vi "Scan_Table_Mode.vi"(0 "Mode":T1) -> (1 "Simulate Mode ?":bool, 2 "Log Full Res Data?":bool, 3 "Minimum Scan Period (ms)":i32)   [LabVIEW 2022 SP3]
uses:
  Anemometry/Anemometry Sub Vis/Controls/Serveds.ctl
  Anemometry/Anemometry Sub Vis/Globals/Constants_global.vi
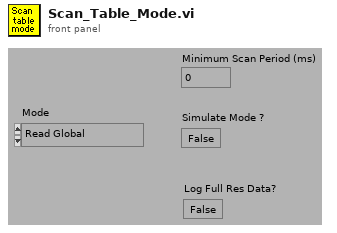
[diagram p1: front panel]
types:
  T1 = typedef "Serveds.ctl" = enum16{"Read Global", "Load Global From File"}
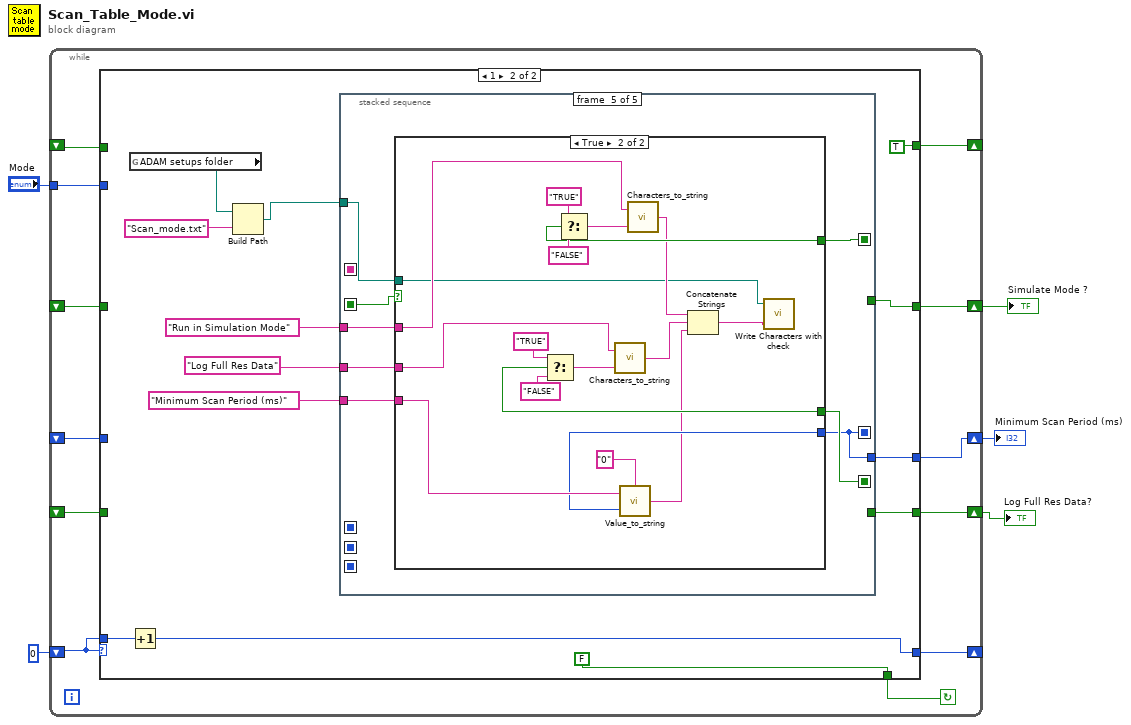
[diagram p0: block diagram]
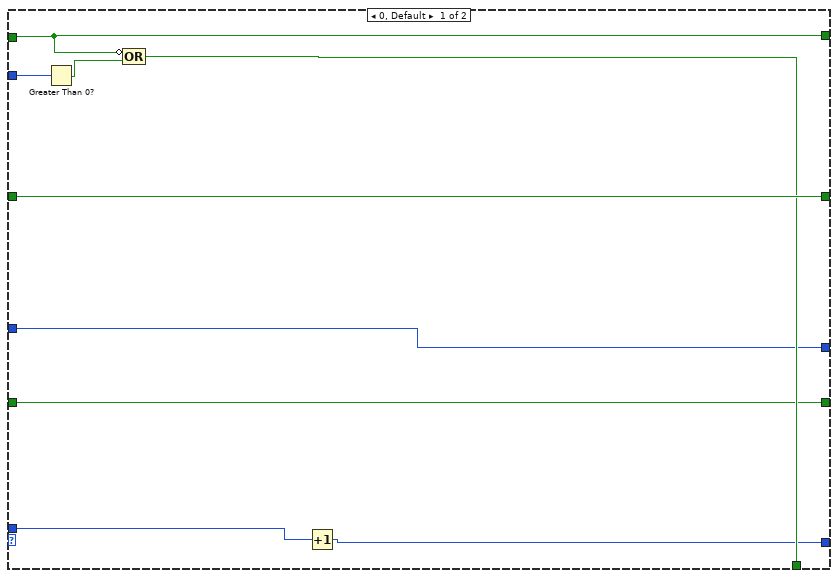
[diagram p2: hidden frame]
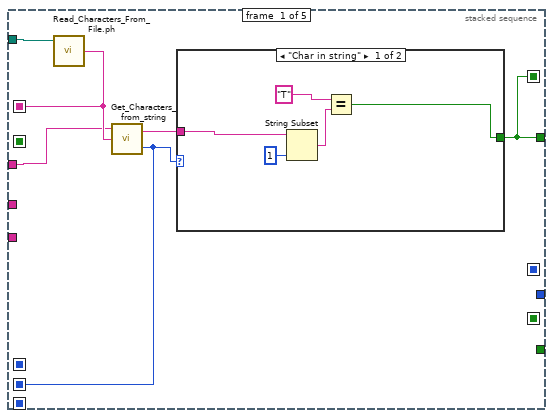
[diagram p3: hidden frame]
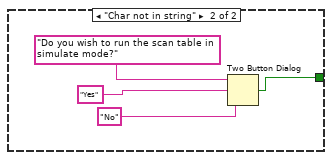
[diagram p4: hidden frame]
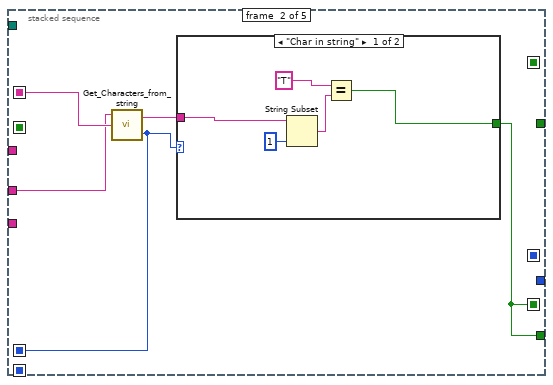
[diagram p5: hidden frame]
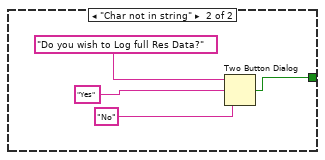
[diagram p6: hidden frame]
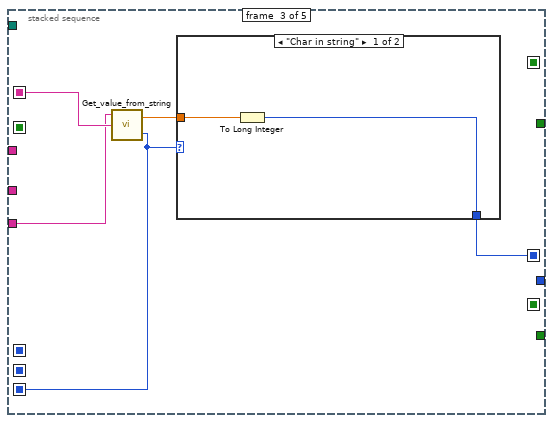
[diagram p7: hidden frame]
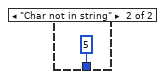
[diagram p8: hidden frame]
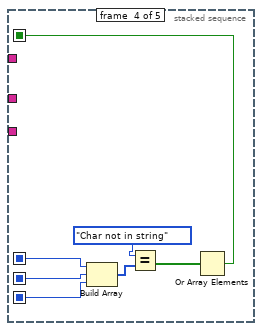
[diagram p9: hidden frame]
diagram:
  n1 = while {
    tunnel: "Mode" -> [w11]
    shift-left: 0 -> [w12]
    shift-right: [w14] -> _
    shift-left: _ -> [w16]
    shift-right: [w13] -> w3
    shift-left: _ -> [w17]
    shift-right: [w10] -> _
    shift-right: [w9] -> w2
    shift-left: _ -> [w8]
    shift-right: [w7] -> w1
    shift-left: _ -> [w6]
    stop <- w15 continue-if-true
    n2 = case shown="1" w12 {
      tunnel: w17 -> [w20 _]
      tunnel: w16 -> [w26 _]
      tunnel: [w23 FALSE] -> w15
      tunnel: [w21 w37] -> w14
      tunnel: [w26 w34] -> w13
      tunnel: w12 -> [w22 w38]
      tunnel: w11 -> [w25 _]
      tunnel: [w20 TRUE] -> w10
      tunnel: [w19 w29] -> w9
      tunnel: w8 -> [w19 _]
      tunnel: [w18 w27] -> w7
      tunnel: w6 -> [w18 _]
      frame 0, Default {
        n3 = Greater Than 0?(x=w25) -> (x > 0?=w24:bool)
        n4 = Compound Arithmetic op=OR(invert w20, w24) -> (w23:bool)
        n5 = Increment(x=w22) -> (x+1=w21:i32)
      }
      frame 1 {
        n6 = global read "Constants_global.vi" "ADAM setups folder"() -> (w36:path)
        n7 = Increment(x=w38) -> (x+1=w37:i32)
        n8 = Build Path(base path=w36, name or relative path="Scan_mode.txt" ("Substring")) -> (appended path=w32:path)
        n9 = stacked-sequence {
          seq-local: [w43 _ _ _ _] -> [_ w58 w72 _ _]
          seq-local: [_ w56 _ _ _] -> [_ _ _ w80 _]
          seq-local: [w41 _ _ _ _] -> [_ _ _ w79 _]
          seq-local: [w40 _ _ _ _] -> [_ _ _ _ w91]
          seq-local: [_ w55 _ _ _] -> [_ _ _ _ w89]
          seq-local: [_ _ w71 _ _] -> [_ _ _ w78 _]
          seq-local: [_ _ w69 _ _] -> [_ _ _ _ w84]
          seq-local: [_ _ _ w77 _] -> [_ _ _ _ w86]
          tunnel: "Run in Simulation Mode" ("character string") -> [w42 _ _ _ w90]
          tunnel: [w40 _ _ _ _] -> w34
          tunnel: [_ w55 _ _ _] -> w29
          tunnel: w32 -> [w44 _ _ _ w88]
          tunnel: "Log Full Res Data" ("character string") -> [_ w57 _ _ w87]
          tunnel: "Minimum Scan Period (ms)" ("character string") -> [_ _ w70 _ w85]
          tunnel: [_ _ _ _ w84] -> w27
          frame #0 {
            n10 = call "Read_Characters_From_File.ph.vi"("file path (dialog if empty)"=w44) -> ("character string"=w43:string)  [unwired: 1 in, 7 out]
            n11 = call "Get_Characters_from_string.vi"("Input string"=w43, "Variable name"=w42) -> ("Status"=w41:enum16{"Char in string", "Char not in string"}, "Value"=w45:string)  [unwired: 1 in]
            n12 = case shown="\"Char in string\"" w41 {
              tunnel: w45 -> [w50 _]
              tunnel: [w46 w51] -> w40
              frame "Char in string" {
                n13 = String Subset(string=w50, length (rest)=1 ("length (rest)")) -> (substring=w48:string)  [unwired: 1 out]
                n14 = Equal?(x="T", y=w48) -> (x = y?=w46:bool)
              }
              frame "Char not in string" {
                n15 = Two Button Dialog(message="Do you wish to run the scan table in simulate mode?", 1:"No" ("F button name (\"Cancel\")"), 2:"Yes" ("T button name (\"OK\")")) -> (T button?=w51:bool)
              }
            }
          }
          frame #1 {
            n16 = call "Get_Characters_from_string.vi"("Input string"=w58, "Variable name"=w57) -> ("Status"=w56:enum16{"Char in string", "Char not in string"}, "Value"=w59:string)  [unwired: 1 in]
            n17 = case shown="\"Char in string\"" w56 {
              tunnel: w59 -> [w64 _]
              tunnel: [w60 w65] -> w55
              frame "Char in string" {
                n18 = String Subset(string=w64, length (rest)=1 ("length (rest)")) -> (substring=w62:string)  [unwired: 1 out]
                n19 = Equal?(x="T", y=w62) -> (x = y?=w60:bool)
              }
              frame "Char not in string" {
                n20 = Two Button Dialog(message="Do you wish to Log full Res Data?", 1:"No" ("F button name (\"Cancel\")"), 2:"Yes" ("T button name (\"OK\")")) -> (T button?=w65:bool)
              }
            }
          }
          frame #2 {
            n21 = call "Get_value_from_string.vi"("Input string"=w72, "Variable name"=w70) -> ("Status"=w71:enum16{"Char in string", "Char not in string"}, "Value"=w73:dbl)  [unwired: 1 in]
            n22 = case shown="\"Char in string\"" w71 {
              tunnel: w73 -> [w75 _]
              tunnel: [w74 5] -> w69
              frame "Char in string" {
                n23 = To Long Integer(number=w75) -> (32bit integer=w74:i32)
              }
              frame "Char not in string" {
              }
            }
          }
          frame #3 {
            n24 = Build Array(w80, w79, w78) -> (w82:enum16{"Char in string", "Char not in string"}[])
            n25 = Equal?(x=enum16{"Char in string", "Char not in string"}."Char not in string" ("Status"), y=w82) -> (x = y?=w81:bool[])
            n26 = Or Array Elements(Boolean array=w81) -> (logical OR=w77:bool)
          }
          frame #4 {
            n27 = case shown="True" w86 {
              tunnel: w91 -> [_ w106]
              tunnel: w90 -> [_ w105]
              tunnel: w89 -> [_ w101]
              tunnel: w87 -> [_ w100]
              tunnel: w88 -> [_ w93]
              tunnel: w85 -> [_ w97]
              tunnel: w84 -> [_ w95]
              frame False {
              }
              frame True {
                n28 = Select(t="TRUE" ("Characters to write"), s=w101, f="FALSE") -> (s? t:f=w102:string)
                n29 = Select(t="TRUE" ("Characters to write"), s=w106, f="FALSE") -> (s? t:f=w109:string)
                n30 = call "Characters_to_string.vi"("Characters to write"=w102, "Label for characters"=w100) -> ("Output string"=w99:string)  [unwired: 1 in]
                n31 = call "Value_to_string.vi"("precision"="0", "Value"=w95, "Label for value"=w97) -> ("Output string"=w94:string)
                n32 = call "Characters_to_string.vi"("Characters to write"=w109, "Label for characters"=w105) -> ("Output string"=w98:string)  [unwired: 1 in]
                n33 = Concatenate Strings(w98, w99, w94) -> (w92:string)
                n34 = call "Write Characters with check.vi"("String to Write"=w92, "file (use dialog)"=w93) -> ()  [unwired: 2 in, 1 out]
              }
            }
          }
        }
      }
    }
  }
  "Simulate Mode ?" <- w3
  "Log Full Res Data?" <- w2
  "Minimum Scan Period (ms)" <- w1
